vi "Execute Single Point Write Request.vi"(8 "error in (no error)":errorcluster, 9 "Write Request":refnum<class "WriteRequest.lvclass">, 10 "Connection ID":string, 11 "MultiplexedConnectionHandler in":refnum<class "MultiplexedConnectionHandler.lvclass">) -> (0 "error out":errorcluster, 3 "MultiplexedConnectionHandler out":refnum<class "MultiplexedConnectionHandler.lvclass">)   [LabVIEW 2020, in "MultiplexedConnectionHandler.lvlib" / "MultiplexedConnectionHandler.lvclass"]
uses:
  <vilib>/gpm_packages/@cs/Network-interface/Source/MultiplexedConnectionHandler/MultiplexedConnectionHandler/MultiplexedConnectionHandler.lvclass
  C:/Program Files/National Instruments/LabVIEW 2020/vi.lib/gpm_packages/@cs/Network-interface/Source/Logged Actor/LoggedActor.lvclass
  C:/Program Files/National Instruments/LabVIEW 2020/vi.lib/gpm_packages/@cs/Network-interface/Source/PersistantConnectionHandler/PersistantConnectionHandler/PersistantConnectionHandler.lvclass
  <vilib>/gpm_packages/@cs/Network-interface/Source/MessagingInterfaces/WriteRequest/WriteRequest.lvclass
  <vilib>/gpm_packages/@cs/Network-interface/Source/MultiplexedConnectionHandler/MultiplexedConnectionHandler/MultiplexedConnectionHandler.lvclass/MultiplexedConnectionHandler.ctl
  <vilib>/gpm_packages/@cs/event-logger/Source/Composed Log/Types/Log Level.ctl
  <vilib>/gpm_packages/@cs/Network-interface/Source/Logged Actor/LoggedActor.lvclass/LoggedActor.ctl
  <vilib>/gpm_packages/@cs/event-logger/Source/Composed Log/LoggerReference/LoggerReference.lvclass/LoggerReference.ctl
  <vilib>/ActorFramework/Message Enqueuer/Message Enqueuer.lvclass
  <vilib>/gpm_packages/@cs/Network-interface/Source/Connection Reference/Connection Reference/Connection Reference.lvclass
  <vilib>/gpm_packages/@cs/event-logger/Source/Composed Log/LoggerReference/Log Event.vi
  <vilib>/gpm_packages/@cs/event-logger/Source/Composed Log/LoggerReference/Log.vi
  <vilib>/gpm_packages/@cs/event-logger/Source/Composed Log/LoggerReference/Get Valid Event Time.vi
  <vilib>/gpm_packages/@cs/event-logger/Source/Composed Log/LoggerReference/Remove Stale Logs.vi
  <vilib>/ErrorRing/Error Ring.xnode
  <vilib>/gpm_packages/@cs/Network-interface/Source/PersistantConnectionHandler/PersistantConnectionHandler/PersistantConnectionHandler.lvclass
  <vilib>/gpm_packages/@cs/Network-interface/Source/Logged Actor/LoggedActor.lvclass
  <vilib>/gpm_packages/@cs/event-logger/Source/Composed Log/Composed Log.lvlib
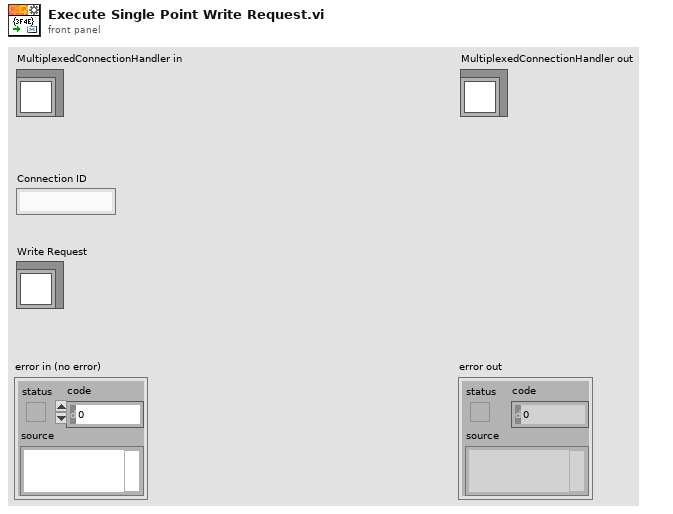
[diagram p1: front panel]
types:
  T1 = typedef "Composed Log.lvlib/Log Level.ctl" = enum16{"Debug", "Info", "Warning", "Error", "Critical"}
  T2 = cluster{"Connection Manager Queue":refnum<class "Message Enqueuer.lvclass">, "Connection Reference":refnum<data-value>}
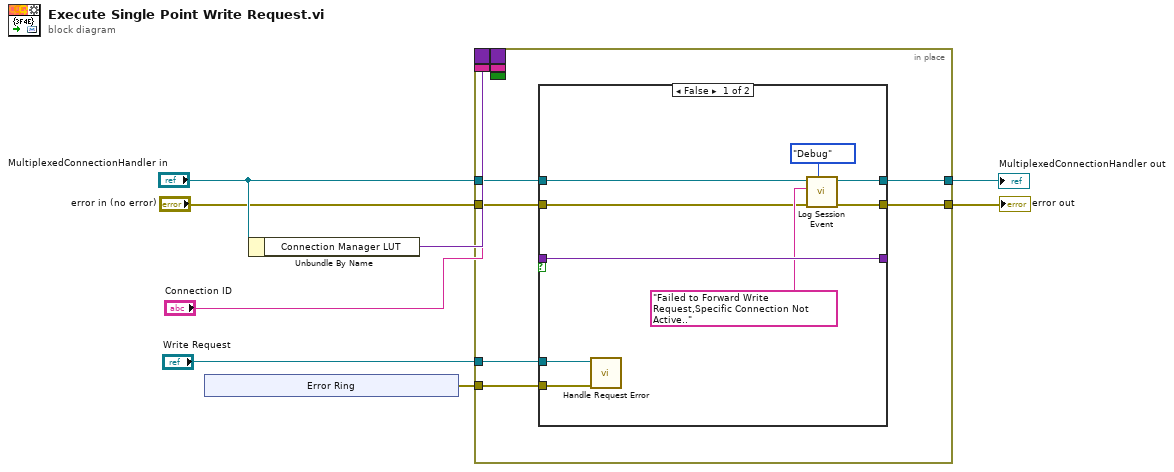
[diagram p0: block diagram]
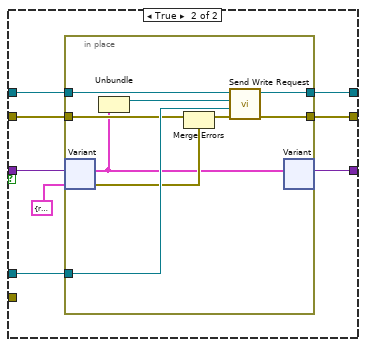
[diagram p2: hidden frame]
diagram:
  n1 = xnode "Error Ring"() -> ("error out"=w1:errorcluster)
  n2 = Unbundle By Name("MultiplexedConnectionHandler in") -> ("Connection Manager LUT"=w3:variant)
  n3 = in-place {
    in-place-border: [w17] -> w8
    in-place-border: "MultiplexedConnectionHandler in" -> [w16]
    in-place-border: "error in (no error)" -> [w15]
    in-place-border: "Write Request" -> [w14]
    in-place-border: [w13] -> w4
    border: w3 -> [_]
    border: "Connection ID" -> [_]
    border: _ -> [_]
    border: _ -> [_]
    border: _ -> [_]
    in-place-border: w1 -> [w9]
    n4 = case shown="False" w10 {
      tunnel: [w18 w33] -> w17
      tunnel: w16 -> [w22 w32]
      tunnel: w15 -> [w20 w31]
      tunnel: w14 -> [w25 w30]
      tunnel: [w19 w29] -> w13
      tunnel: w12 -> [w26 w28]
      tunnel: [w26 w27] -> w11
      tunnel: w9 -> [w24 _]
      frame False {
        n5 = call-dynamic "Handle Request Error.vi"("Request Error"=w24, "WriteRequest in"=w25) -> ()  [unwired: 10 in]
        n6 = call <vilib>:"Log Session Event.vi"("Event Level"=Log_Level."Debug", "error in (no error)"=w20, "Event Data"="Failed to Forward Write Request,Specific Connection Not Active..", "SessionActor in"=w22) -> ("error out"=w19:errorcluster, "SessionActor out"=w18:refnum<class "MultiplexedConnectionHandler.lvclass">)  [unwired: 6 in]
      }
      frame True {
        n7 = in-place {
          in-place-border: w32 -> [w43]
          in-place-border: [w42] -> w33
          in-place-border: w30 -> [w41]
          in-place-border: w31 -> [w40]
          in-place-border: [w39] -> w29
          n8 = in-place-variant #1(w28, T2 {"Connection Manager Queue"=refnum, "Connection Reference"=refnum}) -> (w36:T2, w37:errorcluster)
          n9 = Unbundle(w36) -> ("Connection Manager Queue"=w35:refnum<class "Message Enqueuer.lvclass">)  [unwired: 1 out]
          n10 = Merge Errors(w40, w37) -> (w38:errorcluster)
          n11 = call <vilib>:"Send Write Request.vi"("error in (no error)"=w38, "Write Request"=w41, "Connection Manager Queue"=w35, "PersistantConnectionHandler in"=w43) -> ("error out"=w39:errorcluster, "PersistantConnectionHandler out"=w42:refnum<class "MultiplexedConnectionHandler.lvclass">)  [unwired: 6 in]
          n12 = in-place-variant #1(w36) -> (w27:variant)  [unwired: 1 out]
        }
      }
    }
  }
  "error out" <- w4
  "MultiplexedConnectionHandler out" <- w8
